vi "TheTraaaaash.vi"() -> ()   [LabVIEW 2015]
uses:
  <vilib>/Rock Robotics/WPI/Solenoid/WPI_SolenoidChannel.ctl
  <vilib>/Rock Robotics/WPI/Solenoid/WPI_SolenoidOpenDouble.vi
panel:
  in  "Retract Solenoid Channel 2":T1
  in  "Extend Solenoid Channel 2":T1=enum."Solenoid 1"
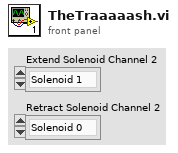
[diagram p1: front panel]
types:
  T1 = typedef "WPI_SolenoidChannel.ctl" = enum8{"Solenoid 0", "Solenoid 1", "Solenoid 2", "Solenoid 3", "Solenoid 4", "Solenoid 5", "Solenoid 6", "Solenoid 7", "Invalid"}
  T2 = typedef "WPI_SolenoidDevRef.ctl" = cluster{"DevStatus":errorcluster, "Pneumatics Control Module":u8, "Forward Solenoid Channel":T1, "Reverse Solenoid Channel":T1}
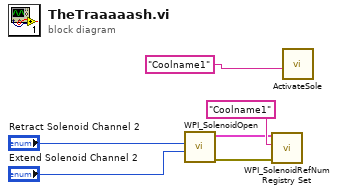
[diagram p0: block diagram]
diagram:
  n1 = call-poly <vilib>:"WPI_SolenoidOpen.vi"("Reverse Solenoid Channel"="Extend Solenoid Channel 2", "Forward Solenoid Channel"="Retract Solenoid Channel 2") -> ("error out"=w3:errorcluster, "SolenoidDevRef"=w4:T2)  [unwired: 2 in, 6 out]
  n2 = call <vilib>:"WPI_SolenoidRefNum Registry Set.vi"("error in (no error)"=w3, "refnum name"="Coolname1", "SolenoidDevRef"=w4) -> ()  [unwired: 7 in, 2 out]
  n3 = call "ActivateSole.vi"("String"="Coolname1") -> ()  [unwired: 11 in]
